vi "User_input.vi"(1 "Main Vi":refnum<vi>, 2 "Speed Threshold (km/h) Ref":refnum<vi>, 3 "Start Ref":refnum<vi>) -> ()   [LabVIEW 2020]
uses:
  <vilib>/Platform/TimedLoop/XDataNode/timing_clust.ctl
  <vilib>/Platform/TimedLoop/XDataNode/nitl_modes.ctl
  <vilib>/Platform/TimedLoop/XDataNode/wakeup.ctl
  <vilib>/platform/TimedLoop/XDataNode/XDataNode.xnode
  <vilib>/Platform/TimedLoop/XDataNode/XDNodeRunTimeDep.lvlib
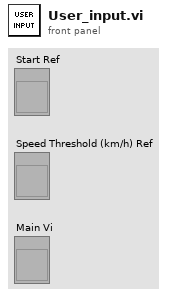
[diagram p1: front panel]
types:
  T1 = enum8{"Enabled", "Disabled", "Disabled and Grayed Out"}
  T2 = typedef "XDNodeRunTimeDep.lvlib/timing_clust.ctl" = cluster{"Expected End [f-1]":u64, "Actual End [f-1]":u64, "Finished Late? [f-1]":bool, "Expected End [i-1]":u64, "Actual End [i-1]":u64, "Finished Late? [i-1]":bool, "Expected Start [i]":u64, "Actual Start [i]":u64, "Expected Start [f]":u64, "Actual Start [f]":u64, "Source Name":string, "Structure Name":string, "Period":i64, "Deadline":i64, "Offset":i64, "Start":i64, "Priority":i32, "Timeout":i32, "Mode":T3, "Wakeup Reason":T4, "Error":errorcluster, "Source Type":string, "Secondary Source Type":string, "Global End Time":u64, "Global Start Time":u64, "Frame Duration":u64, "Iteration Duration":u64, "Assigned CPU":i32, "I/O Scan Engine Mode":u32}
  T3 = typedef "XDNodeRunTimeDep.lvlib/nitl_modes.ctl" = enum32{"No Change", "Process missed periods, maintain original phase", "Discard missed periods, maintain original phase", "Process missed periods, ignore original phase", "Discard missed periods, ignore original phase"}
  T4 = typedef "XDNodeRunTimeDep.lvlib/wakeup.ctl" = enum32{"Normal", "Aborted", "Asynchronous wakeup", "Timing source error", "Timed loop error", "Timeout"}
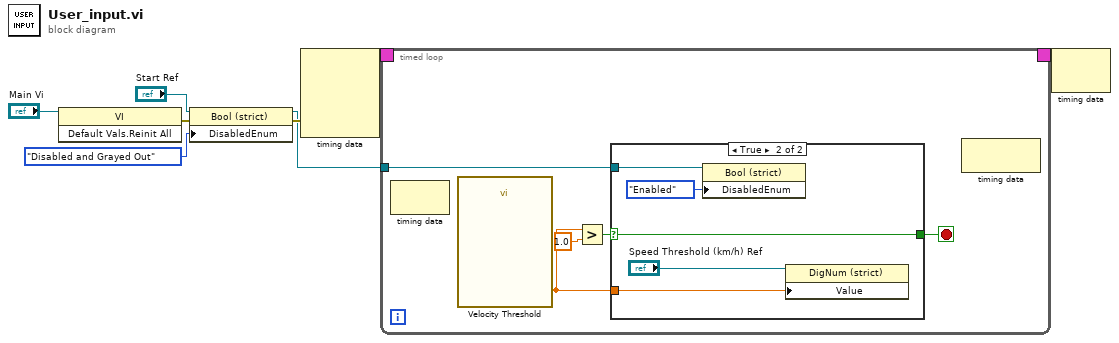
[diagram p0: block diagram]
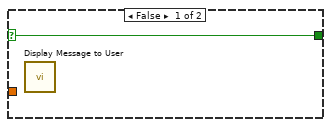
[diagram p2: hidden frame]
diagram:
  n1 = invoke class="VI" method="Default Vals.Reinit All"(reference="Main Vi") -> (error out=w3:errorcluster)  [unwired: 2 in, 2 out]
  n2 = property on="Property Node" class="Bool (strict)"(reference="Start Ref", error in=w3, "DisabledEnum"=T1."Disabled and Grayed Out" ("Disabled")) -> (reference out=w1:refnum<vi>, error out=w5:errorcluster)
  n3 = node-c288(w5) -> (w8:T2)  [unwired: 3 in]
  n4 = timed-loop {
    timing: w8 -> [_]
    timing-out: [_] -> w7
    tunnel: w1 -> [w9]
    stop <- w11 stop-if-true
    n5 = node-c288() -> ()  [unwired: 1 in, 1 out]
    n6 = call "Velocity Threshold"() -> ("velocity"=w10:dbl)  [unwired: 17 in, 2 out]
    n7 = Greater?(x=w10, y=1.0) -> (0:w12:bool)
    n8 = case shown="True" w12 {
      selector: w12 -> [w14 w19]
      tunnel: [w14 w19] -> w11
      tunnel: w10 -> [_ w17]
      tunnel: w9 -> [_ w15]
      frame False {
        n9 = call "Display Message to User"() -> ()  [unwired: 10 in, 2 out]
      }
      frame True {
        n10 = property on="Property Node" class="Bool (strict)"(reference=w15, "DisabledEnum"=T1."Enabled" ("Disabled")) -> ()  [unwired: 1 in, 2 out]
        n11 = property on="Property Node" class="DigNum (strict)"(reference="Speed Threshold (km/h) Ref", "Value"=w17) -> ()  [unwired: 1 in, 2 out]
      }
    }
    n12 = node-c288() -> ()  [unwired: 1 in, 1 out]
  }
  n13 = node-c288(w7) -> ()  [unwired: 1 out]
